vi "country.vi"(8 "Error In":errorcluster, 11 "QLocale In":refnum<class "QLocale.lvclass">) -> (0 "Error Out":errorcluster, 2 "Value":T1 items=["AnyCountry", "Afghanistan", "Albania", "Algeria", "AmericanSamoa", "Andorra", "Angola", "Anguilla", "Antarctica", "AntiguaAndBarbuda", "Argentina", "Armenia", "Aruba", "Australia", "Austria", "Azerbaijan", "Bahamas", "Bahrain", "Bangladesh", "Barbados", "Belarus", "Belgium", "Belize", "Benin", "Bermuda", "Bhutan", "Bolivia", "BosniaAndHerzegowina", "Botswana", "BouvetIsland", "Brazil", "BritishIndianOceanTerritory", "Brunei", "Bulgaria", "BurkinaFaso", "Burundi", "Cambodia", "Cameroon", "Canada", "CapeVerde", "CaymanIslands", "CentralAfricanRepublic", "Chad", "Chile", "China", "ChristmasIsland", "CocosIslands", "Colombia", "Comoros", "CongoKinshasa", "CongoBrazzaville", "CookIslands", "CostaRica", "IvoryCoast", "Croatia", "Cuba", "Cyprus", "CzechRepublic", "Denmark", "Djibouti", "Dominica", "DominicanRepublic", "EastTimor", "Ecuador", "Egypt", "ElSalvador", "EquatorialGuinea", "Eritrea", "Estonia", "Ethiopia", "FalklandIslands", "FaroeIslands", "Fiji", "Finland", "France", "Guernsey", "FrenchGuiana", "FrenchPolynesia", "FrenchSouthernTerritories", "Gabon", "Gambia", "Georgia", "Germany", "Ghana", "Gibraltar", "Greece", "Greenland", "Grenada", "Guadeloupe", "Guam", "Guatemala", "Guinea", "GuineaBissau", "Guyana", "Haiti", "HeardAndMcDonaldIslands", "Honduras", "HongKong", "Hungary", "Iceland", "India", "Indonesia", "Iran", "Iraq", "Ireland", "Israel", "Italy", "Jamaica", "Japan", "Jordan", "Kazakhstan", "Kenya", "Kiribati", "NorthKorea", "SouthKorea", "Kuwait", "Kyrgyzstan", "Laos", "Latvia", "Lebanon", "Lesotho", "Liberia", "Libya", "Liechtenstein", "Lithuania", "Luxembourg", "Macau", "Macedonia", "Madagascar", "Malawi", "Malaysia", "Maldives", "Mali", "Malta", "MarshallIslands", "Martinique", "Mauritania", "Mauritius", "Mayotte", "Mexico", "Micronesia", "Moldova", "Monaco", "Mongolia", "Montserrat", "Morocco", "Mozambique", "Myanmar", "Namibia", "NauruCountry", "Nepal", "Netherlands", "CuraSao", "NewCaledonia", "NewZealand", "Nicaragua", "Niger", "Nigeria", "Niue", "NorfolkIsland", "NorthernMarianaIslands", "Norway", "Oman", "Pakistan", "Palau", "PalestinianTerritories", "Panama", "PapuaNewGuinea", "Paraguay", "Peru", "Philippines", "Pitcairn", "Poland", "Portugal", "PuertoRico", "Qatar", "Reunion", "Romania", "Russia", "Rwanda", "SaintKittsAndNevis", "SaintLucia", "SaintVincentAndTheGrenadines", "Samoa", "SanMarino", "SaoTomeAndPrincipe", "SaudiArabia", "Senegal", "Seychelles", "SierraLeone", "Singapore", "Slovakia", "Slovenia", "SolomonIslands", "Somalia", "SouthAfrica", "SouthGeorgiaAndTheSouthSandwichIslands", "Spain", "SriLanka", "SaintHelena", "SaintPierreAndMiquelon", "Sudan", "Suriname", "SvalbardAndJanMayenIslands", "Swaziland", "Sweden", "Switzerland", "Syria", "Taiwan", "Tajikistan", "Tanzania", "Thailand", "Togo", "TokelauCountry", "Tonga", "TrinidadAndTobago", "Tunisia", "Turkey", "Turkmenistan", "TurksAndCaicosIslands", "TuvaluCountry", "Uganda", "Ukraine", "UnitedArabEmirates", "UnitedKingdom", "UnitedStates", "UnitedStatesMinorOutlyingIslands", "Uruguay", "Uzbekistan", "Vanuatu", "VaticanCityState", "Venezuela", "Vietnam", "BritishVirginIslands", "UnitedStatesVirginIslands", "WallisAndFutunaIslands", "WesternSahara", "Yemen", "CanaryIslands", "Zambia", "Zimbabwe", "ClippertonIsland", "Montenegro", "Serbia", "SaintBarthelemy", "SaintMartin", "LatinAmerica", "AscensionIsland", "AlandIslands", "DiegoGarcia", "CeutaAndMelilla", "IsleOfMan", "Jersey", "TristanDaCunha", "SouthSudan", "Bonaire", "SintMaarten", "Kosovo", "EuropeanUnion", "OutlyingOceania", "World", "Europe"], 3 "QLocale Out":refnum<class "QLocale.lvclass">)   [LabVIEW 2014, in "QLocale.lvclass"]
doc: "LabVIEW-specific documentation is not yet available. See <b>https://doc.qt.io/qt-5/qlocale.html#country</b>"
uses:
  QLocale.lvclass
  Country.ctl
  LQSerialData/LQSerialData.lvclass/LQSerialData.ctl
  LQ Core.lvlib
  LQSerialData/LQSerialData.lvclass
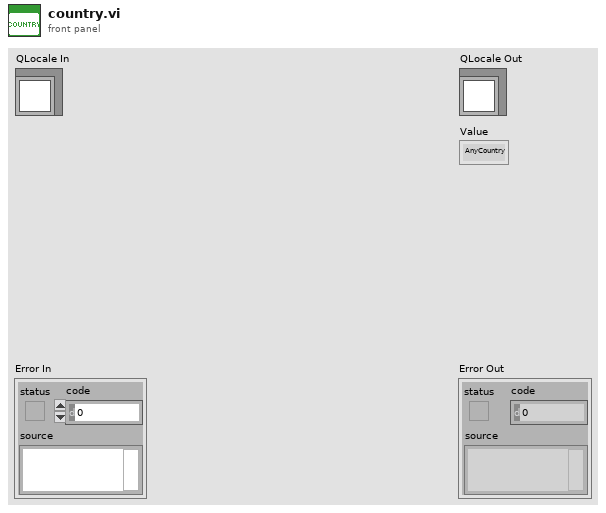
[diagram p1: front panel]
types:
  T1 = typedef "QLocale.lvclass/Country.ctl" = i32
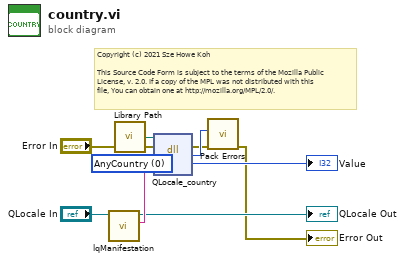
[diagram p0: block diagram]
diagram:
  w8 = T1 0 items=["AnyCountry", "Afghanistan", "Albania", "Algeria", "AmericanSamoa", "Andorra", "Angola", "Anguilla", "Antarctica", "AntiguaAndBarbuda", "Argentina", "Armenia", "Aruba", "Australia", "Austria", "Azerbaijan", "Bahamas", "Bahrain", "Bangladesh", "Barbados", "Belarus", "Belgium", "Belize", "Benin", "Bermuda", "Bhutan", "Bolivia", "BosniaAndHerzegowina", "Botswana", "BouvetIsland", "Brazil", "BritishIndianOceanTerritory", "Brunei", "Bulgaria", "BurkinaFaso", "Burundi", "Cambodia", "Cameroon", "Canada", "CapeVerde", "CaymanIslands", "CentralAfricanRepublic", "Chad", "Chile", "China", "ChristmasIsland", "CocosIslands", "Colombia", "Comoros", "CongoKinshasa", "CongoBrazzaville", "CookIslands", "CostaRica", "IvoryCoast", "Croatia", "Cuba", "Cyprus", "CzechRepublic", "Denmark", "Djibouti", "Dominica", "DominicanRepublic", "EastTimor", "Ecuador", "Egypt", "ElSalvador", "EquatorialGuinea", "Eritrea", "Estonia", "Ethiopia", "FalklandIslands", "FaroeIslands", "Fiji", "Finland", "France", "Guernsey", "FrenchGuiana", "FrenchPolynesia", "FrenchSouthernTerritories", "Gabon", "Gambia", "Georgia", "Germany", "Ghana", "Gibraltar", "Greece", "Greenland", "Grenada", "Guadeloupe", "Guam", "Guatemala", "Guinea", "GuineaBissau", "Guyana", "Haiti", "HeardAndMcDonaldIslands", "Honduras", "HongKong", "Hungary", "Iceland", "India", "Indonesia", "Iran", "Iraq", "Ireland", "Israel", "Italy", "Jamaica", "Japan", "Jordan", "Kazakhstan", "Kenya", "Kiribati", "NorthKorea", "SouthKorea", "Kuwait", "Kyrgyzstan", "Laos", "Latvia", "Lebanon", "Lesotho", "Liberia", "Libya", "Liechtenstein", "Lithuania", "Luxembourg", "Macau", "Macedonia", "Madagascar", "Malawi", "Malaysia", "Maldives", "Mali", "Malta", "MarshallIslands", "Martinique", "Mauritania", "Mauritius", "Mayotte", "Mexico", "Micronesia", "Moldova", "Monaco", "Mongolia", "Montserrat", "Morocco", "Mozambique", "Myanmar", "Namibia", "NauruCountry", "Nepal", "Netherlands", "CuraSao", "NewCaledonia", "NewZealand", "Nicaragua", "Niger", "Nigeria", "Niue", "NorfolkIsland", "NorthernMarianaIslands", "Norway", "Oman", "Pakistan", "Palau", "PalestinianTerritories", "Panama", "PapuaNewGuinea", "Paraguay", "Peru", "Philippines", "Pitcairn", "Poland", "Portugal", "PuertoRico", "Qatar", "Reunion", "Romania", "Russia", "Rwanda", "SaintKittsAndNevis", "SaintLucia", "SaintVincentAndTheGrenadines", "Samoa", "SanMarino", "SaoTomeAndPrincipe", "SaudiArabia", "Senegal", "Seychelles", "SierraLeone", "Singapore", "Slovakia", "Slovenia", "SolomonIslands", "Somalia", "SouthAfrica", "SouthGeorgiaAndTheSouthSandwichIslands", "Spain", "SriLanka", "SaintHelena", "SaintPierreAndMiquelon", "Sudan", "Suriname", "SvalbardAndJanMayenIslands", "Swaziland", "Sweden", "Switzerland", "Syria", "Taiwan", "Tajikistan", "Tanzania", "Thailand", "Togo", "TokelauCountry", "Tonga", "TrinidadAndTobago", "Tunisia", "Turkey", "Turkmenistan", "TurksAndCaicosIslands", "TuvaluCountry", "Uganda", "Ukraine", "UnitedArabEmirates", "UnitedKingdom", "UnitedStates", "UnitedStatesMinorOutlyingIslands", "Uruguay", "Uzbekistan", "Vanuatu", "VaticanCityState", "Venezuela", "Vietnam", "BritishVirginIslands", "UnitedStatesVirginIslands", "WallisAndFutunaIslands", "WesternSahara", "Yemen", "CanaryIslands", "Zambia", "Zimbabwe", "ClippertonIsland", "Montenegro", "Serbia", "SaintBarthelemy", "SaintMartin", "LatinAmerica", "AscensionIsland", "AlandIslands", "DiegoGarcia", "CeutaAndMelilla", "IsleOfMan", "Jersey", "TristanDaCunha", "SouthSudan", "Bonaire", "SintMaarten", "Kosovo", "EuropeanUnion", "OutlyingOceania", "World", "Europe"] ("retVal")
  # "Copyright (c) 2021 Sze Howe Koh\n\nThis Source Code Form is subject to the terms of the Mozilla Public\nLicense, v. 2.0. If a copy of the MPL was not distributed with this\nfile, You can obtain one at http://mozilla.org/MPL/2.0/."
  n1 = call "lqManifestation.vi"("LQSerialData in"="QLocale In") -> ("Manifestation"=w7:string, "LQSerialData out"=→"QLocale Out":refnum<class "QLocale.lvclass">)  [unwired: 9 in]
  n2 = call "Library Path.vi"() -> ("Library Path"=w4:path)
  n3 = dll-call lib="?" fn="QLocale_country"(path in=w4, error in="Error In", "_retVal"=w8, "_instance"=w7) -> (error out=w2:errorcluster, w3:i32, "_retVal"=→"Value":i32)  [unwired: 2 in, 1 out]
  n4 = call "Pack Errors.vi"("Error In"=w2, "Error Code"=w3) -> ("Error Out"=→"Error Out":errorcluster)  [unwired: 9 in]
